vi "3.Dashboard.vi"() -> ()   [LabVIEW 2023]
uses:
  UnderAutomation.UniversalRobots/UnderAutomation.UniversalRobots.lvlib
  C:/Users/fg/Documents/UniversalRobots.vi/LabVIEW_2024/UnderAutomation.UniversalRobots/lib/UnderAutomation.UniversalRobots.dll
  LabVIEW_2024/UnderAutomation.UniversalRobots/lib/UnderAutomation.UniversalRobots.dll
panel:
  out "Dashboard":refnum<k24>
  out "UR Robot":refnum<k24>
  out "Connected":bool
  in  "Tab Control":enum32{"Connect to robot", "Commands", "State"}(tab)
  in  "Disconnect":bool
  in  "Test":bool
  in  "Key":string
  in  "Licensee":string
  in  "Connect":bool
  in  "IP":string caption="Robot IP Address"
  out "License state":string
  out "Connect error":string
  in  "Release brake":bool
  in  "Power Off":bool
  in  "Power On":bool
  out "Response":cluster{"Message":string, "Succeed":bool}
  in  "Program name":string
  in  "LoadProgram":bool
  in  "Get loaded program":bool
  out "Loaded program":string
  in  "Play":bool
  in  "Pause":bool
  in  "Stop":bool
  in  "Installation":string
  in  "Load installation":bool
  in  "Show popup":bool
  in  "message":string
  in  "Close popup":bool
  in  "Is program saved":bool
  out "IsSaved":bool
  in  "Get program state":bool
  out "Name":string
  out "State":i32(ring) items=["Stopped", "Playing", "Paused"]
  out "Value":T1
  in  "Get variable value":bool
  in  "name":string
  out "remote":bool
  in  "Is in remote control":bool
  in  "Get Serial number":bool
  in  "Get robot mode":bool
  out "Mode":i32(ring) items=["Disconnected"=0, "ConfirmSafety"=1, "Booting"=2, "PowerOff"=3, "PowerOn"=4, "Idle"=5, "BackDrive"=6, "Running"=7, "UpdatingFirmware"=8, "Other"=-1]
  in  "Get robot model":bool
  out "Model":i32(ring)=1 items=["UR5"=1, "UR10"=2, "UR3"=3, "UR16"=4]
  out "SN":string
  in  "stop":bool
  # "UnderAutomation"
  # "https://underautomation.com/universal-robots"
  # "+"
  # "LabVIEW demo app for remote control and monitoring of your Universal Robots cobot"
  # "Connect to robot"
  # "2. Ensure you have a trial or lifetime valid license"
  # "1. Set UR cobot address"
  # "This is a commercial library, you have a 30-day trial period. But you can use it forever if you buy a perpetual licence for your company (regardless of the number of robot, applications or developers)."
  # "If you have a license :"
  # "2. Connect to the robot"
  # "Power"
  # "Program"
  # "Installation"
  # "Popup"
  # "Remote control"
  # "Mode"
  # "Variable"
  # "S/N"
  # "Model"
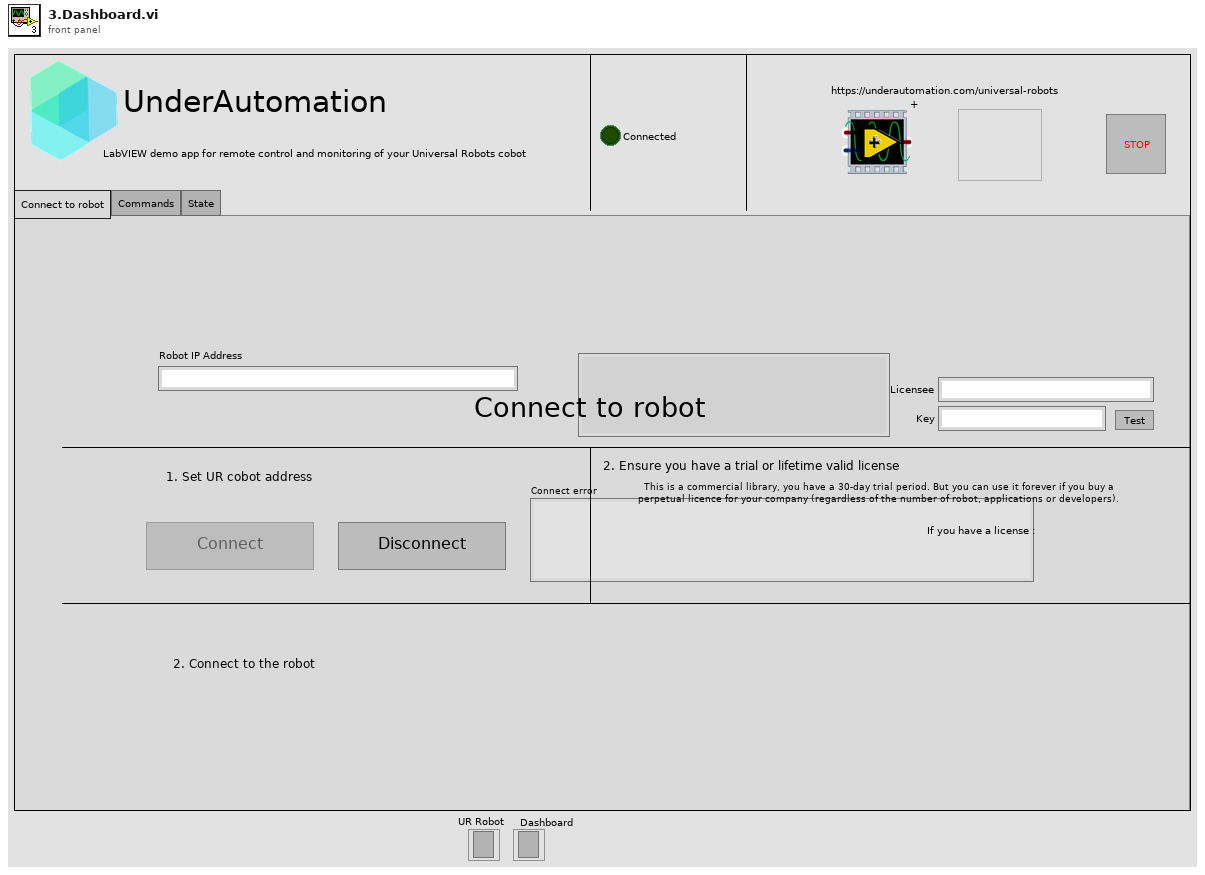
[diagram p1: front panel]
types:
  T1 = cluster{"Name":string, "Milliseconds":i32, "Type":i32, "BoolValue":bool, "FloatValue":sgl, "IntValue":i32, "StringValue":string, "PoseValue":cluster{"X":dbl, "Y":dbl, "Z":dbl, "Rx":dbl, "Ry":dbl, "Rz":dbl}}
  T2 = enum8{"Enabled", "Disabled", "Disabled and Grayed Out"}
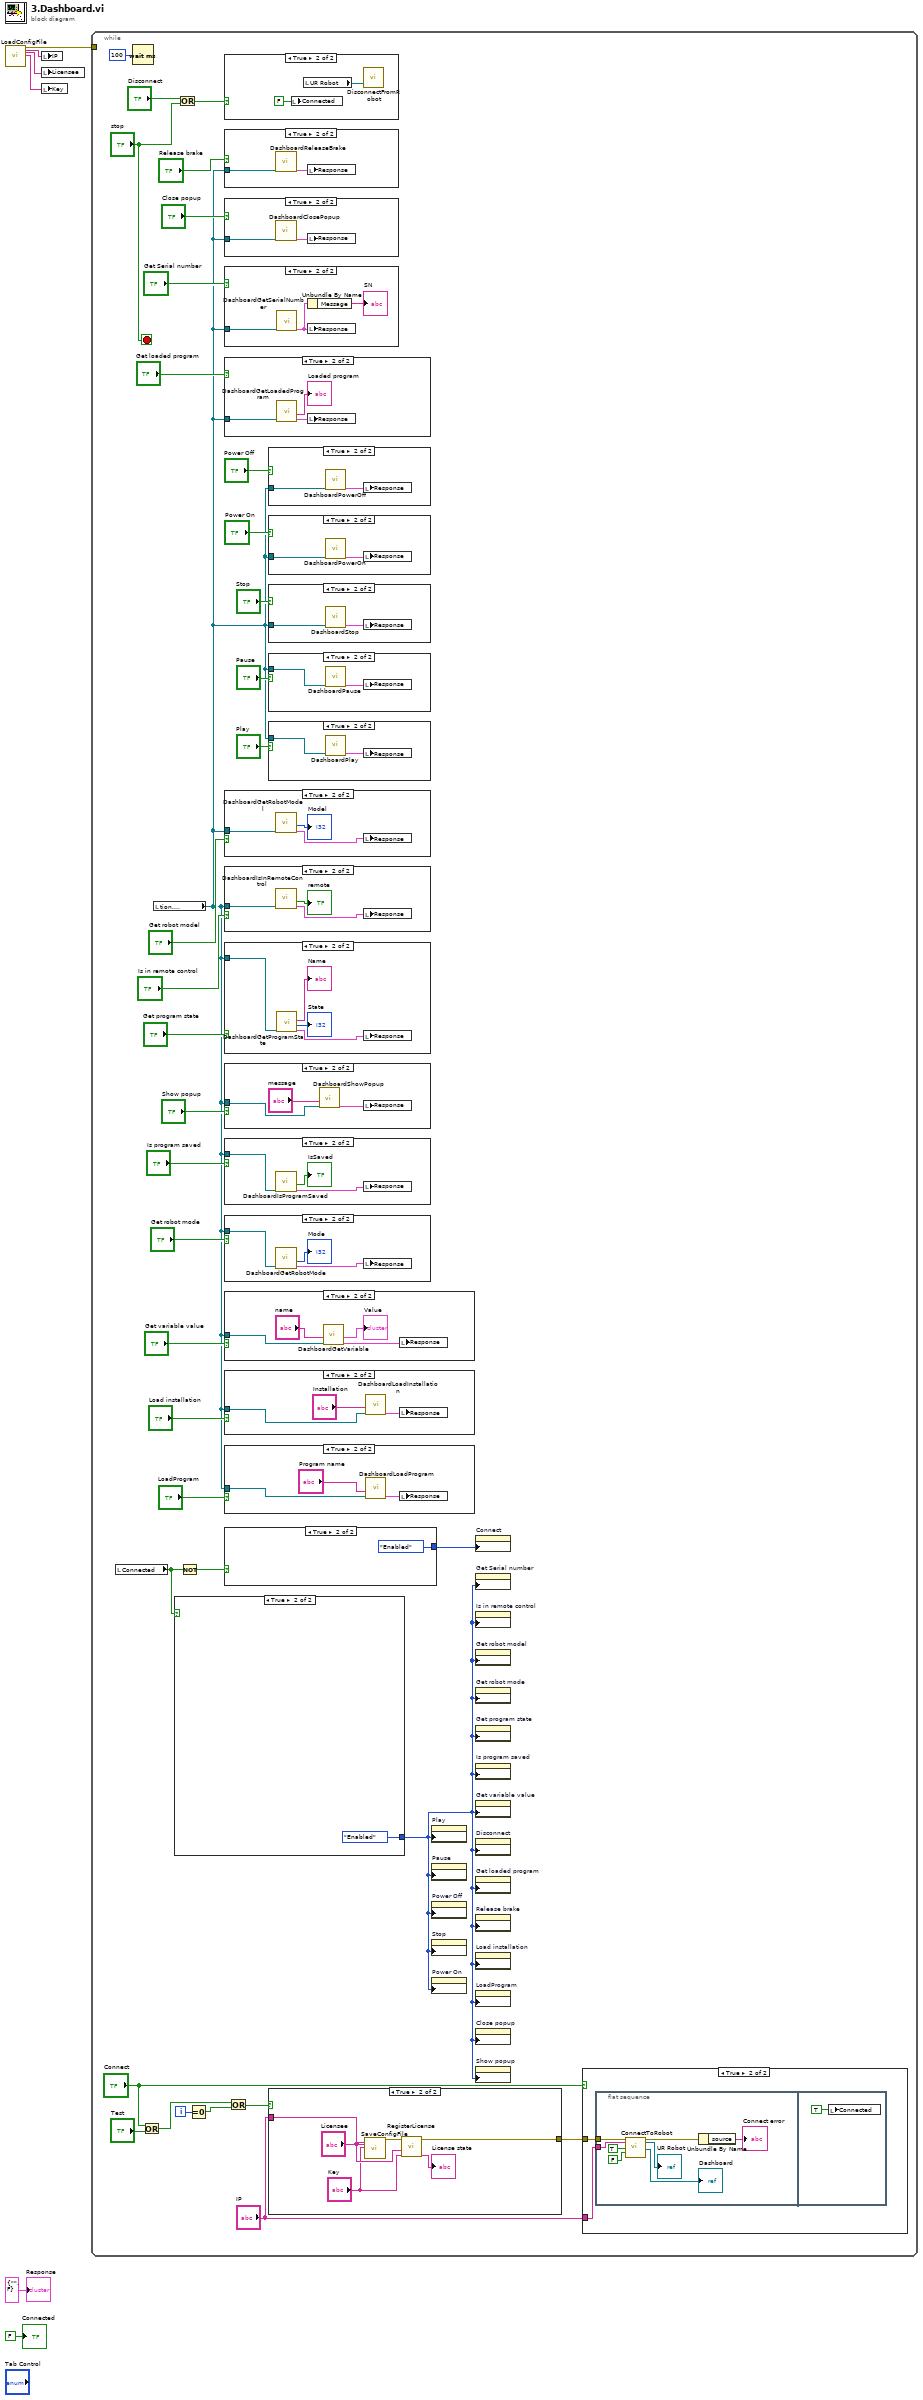
[diagram p0: block diagram]
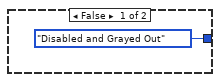
[diagram p20: hidden frame]
diagram:
  n1 = call "LoadConfigFile.vi"() -> ("error out"=w3:errorcluster, "IP"=w4:string, "Licensee"=w6:string, "Key"=w5:string)  [unwired: 22 in, 2 out]
  n2 = local write "IP"(w4) -> ()
  n3 = local write "Licensee"(w6) -> ()
  n4 = local write "Key"(w5) -> ()
  n5 = while {
    tunnel: w3 -> [_]
    i -> [w35]
    stop <- "stop" stop-if-true
    n6 = local read "Connected"() -> (w27:bool)
    n7 = Wait (ms)(milliseconds to wait=u32 100) -> ()  [unwired: 1 out]
    n8 = Or(x="Connect", y="Test") -> (x .or. y?=w33:bool)
    n9 = local read "Dashboard"() -> (w8:refnum<k24>)
    n10 = case shown="True" w27 {
      tunnel: [T2."Disabled and Grayed Out" ("Disabled") T2."Enabled" ("Disabled")] -> w7
      frame False {
      }
      frame True {
      }
    }
    n11 = Or(x="Disconnect", y="stop") -> (x .or. y?=w39:bool)
    n12 = Not(x=w27) -> (.not. x?=w29:bool)
    n13 = Equal To 0?(x=w35) -> (x = 0?=w34:bool)
    n14 = case shown="True" w39 {
      frame False {
      }
      frame True {
        n15 = local write "Connected"(FALSE ("Connected")) -> ()
        n16 = local read "UR Robot"() -> (w114:refnum<k24>)
        n17 = call "DisconnectFromRobot.vi"("UR Robot"=w114) -> ()  [unwired: 2 in, 1 out]
      }
    }
    n18 = case shown="True" "Release brake" {
      tunnel: w8 -> [_ w85]
      frame False {
      }
      frame True {
        n19 = call "DashboardReleaseBrake.vi"("Dashboard"=w85) -> ("Response"=w86:cluster{"Message":string, "Succeed":bool})  [unwired: 9 in, 1 out]
        n20 = local write "Response"(w86) -> ()
      }
    }
    n21 = case shown="True" "Close popup" {
      tunnel: w8 -> [_ w66]
      frame False {
      }
      frame True {
        n22 = call "DashboardClosePopup.vi"("Dashboard"=w66) -> ("Response"=w65:cluster{"Message":string, "Succeed":bool})  [unwired: 9 in, 1 out]
        n23 = local write "Response"(w65) -> ()
      }
    }
    n24 = case shown="True" "Get Serial number" {
      tunnel: w8 -> [_ w64]
      frame False {
      }
      frame True {
        n25 = call "DashboardGetSerialNumber.vi"("Dashboard"=w64) -> ("Response"=w63:cluster{"Message":string, "Succeed":bool})  [unwired: 9 in, 1 out]
        n26 = Unbundle By Name(w63) -> ("Message"=→"SN":string)
        n27 = local write "Response"(w63) -> ()
      }
    }
    n28 = case shown="True" "Get loaded program" {
      tunnel: w8 -> [_ w75]
      frame False {
      }
      frame True {
        n29 = call "DashboardGetLoadedProgram.vi"("Dashboard"=w75) -> ("Response"=w74:cluster{"Message":string, "Succeed":bool}, "loaded program"=→"Loaded program":string)  [unwired: 8 in, 1 out]
        n30 = local write "Response"(w74) -> ()
      }
    }
    n31 = case shown="True" "Get robot model" {
      tunnel: w8 -> [_ w56]
      frame False {
      }
      frame True {
        n32 = call "DashboardGetRobotModel.vi"("Dashboard"=w56) -> ("Response"=w58:cluster{"Message":string, "Succeed":bool}, "Model"=→"Model":i32)  [unwired: 8 in, 1 out]
        n33 = local write "Response"(w58) -> ()
      }
    }
    n34 = case shown="True" "Is in remote control" {
      tunnel: w8 -> [_ w50]
      frame False {
      }
      frame True {
        n35 = call "DashboardIsInRemoteControl.vi"("Dashboard"=w50) -> ("Response"=w52:cluster{"Message":string, "Succeed":bool}, "remote"=→"remote":bool)  [unwired: 8 in, 1 out]
        n36 = local write "Response"(w52) -> ()
      }
    }
    n37 = case shown="True" "Get program state" {
      tunnel: w8 -> [_ w42]
      frame False {
      }
      frame True {
        n38 = call "DashboardGetProgramState.vi"("Dashboard"=w42) -> ("Response"=w45:cluster{"Message":string, "Succeed":bool}, "State"=→"State":i32, "Name"=→"Name":string)  [unwired: 7 in, 1 out]
        n39 = local write "Response"(w45) -> ()
      }
    }
    n40 = case shown="True" "Show popup" {
      tunnel: w8 -> [_ w69]
      frame False {
      }
      frame True {
        n41 = call "DashboardShowPopup.vi"("Dashboard"=w69, "message"="message") -> ("Response"=w68:cluster{"Message":string, "Succeed":bool})  [unwired: 8 in, 1 out]
        n42 = local write "Response"(w68) -> ()
      }
    }
    n43 = case shown="True" "Is program saved" {
      tunnel: w8 -> [_ w53]
      frame False {
      }
      frame True {
        n44 = call "DashboardIsProgramSaved.vi"("Dashboard"=w53) -> ("Response"=w55:cluster{"Message":string, "Succeed":bool}, "IsSaved"=→"IsSaved":bool)  [unwired: 7 in, 2 out]
        n45 = local write "Response"(w55) -> ()
      }
    }
    n46 = case shown="True" "Get robot mode" {
      tunnel: w8 -> [_ w59]
      frame False {
      }
      frame True {
        n47 = call "DashboardGetRobotMode.vi"("Dashboard"=w59) -> ("Response"=w61:cluster{"Message":string, "Succeed":bool}, "Mode"=→"Mode":i32)  [unwired: 8 in, 1 out]
        n48 = local write "Response"(w61) -> ()
      }
    }
    n49 = case shown="True" "Get variable value" {
      tunnel: w8 -> [_ w47]
      frame False {
      }
      frame True {
        n50 = call "DashboardGetVariable.vi"("Dashboard"=w47, "name"="name") -> ("Response"=w49:cluster{"Message":string, "Succeed":bool}, "Value"=→"Value":T1)  [unwired: 7 in, 1 out]
        n51 = local write "Response"(w49) -> ()
      }
    }
    n52 = case shown="True" "Load installation" {
      tunnel: w8 -> [_ w71]
      frame False {
      }
      frame True {
        n53 = call "DashboardLoadInstallation.vi"("Dashboard"=w71, "installation"="Installation") -> ("Response"=w72:cluster{"Message":string, "Succeed":bool})  [unwired: 8 in, 1 out]
        n54 = local write "Response"(w72) -> ()
      }
    }
    n55 = case shown="True" "LoadProgram" {
      tunnel: w8 -> [_ w84]
      frame False {
      }
      frame True {
        n56 = call "DashboardLoadProgram.vi"("Dashboard"=w84, "programName"="Program name") -> ("Response"=w83:cluster{"Message":string, "Succeed":bool})  [unwired: 8 in, 1 out]
        n57 = local write "Response"(w83) -> ()
      }
    }
    n58 = case shown="True" w29 {
      tunnel: [T2."Disabled and Grayed Out" ("Disabled") T2."Enabled" ("Disabled")] -> w28
      frame False {
      }
      frame True {
      }
    }
    n59 = Or(x=w33, y=w34) -> (x .or. y?=w32:bool)
    n60 = case shown="True" "Power Off" {
      tunnel: w8 -> [_ w87]
      frame False {
      }
      frame True {
        n61 = call "DashboardPowerOff.vi"("Dashboard"=w87) -> ("Response"=w88:cluster{"Message":string, "Succeed":bool})  [unwired: 9 in, 1 out]
        n62 = local write "Response"(w88) -> ()
      }
    }
    n63 = case shown="True" "Power On" {
      tunnel: w8 -> [_ w89]
      frame False {
      }
      frame True {
        n64 = call "DashboardPowerOn.vi"("Dashboard"=w89) -> ("Response"=w90:cluster{"Message":string, "Succeed":bool})  [unwired: 9 in, 1 out]
        n65 = local write "Response"(w90) -> ()
      }
    }
    n66 = case shown="True" "Stop" {
      tunnel: w8 -> [_ w77]
      frame False {
      }
      frame True {
        n67 = call "DashboardStop.vi"("Dashboard"=w77) -> ("Response"=w76:cluster{"Message":string, "Succeed":bool})  [unwired: 9 in, 1 out]
        n68 = local write "Response"(w76) -> ()
      }
    }
    n69 = case shown="True" "Pause" {
      tunnel: w8 -> [_ w79]
      frame False {
      }
      frame True {
        n70 = call "DashboardPause.vi"("Dashboard"=w79) -> ("Response"=w78:cluster{"Message":string, "Succeed":bool})  [unwired: 9 in, 1 out]
        n71 = local write "Response"(w78) -> ()
      }
    }
    n72 = case shown="True" "Play" {
      tunnel: w8 -> [_ w81]
      frame False {
      }
      frame True {
        n73 = call "DashboardPlay.vi"("Dashboard"=w81) -> ("Response"=w80:cluster{"Message":string, "Succeed":bool})  [unwired: 9 in, 1 out]
        n74 = local write "Response"(w80) -> ()
      }
    }
    n75 = case shown="True" w32 {
      tunnel: [errorcluster {"status"=FALSE, "code"=0, "source"=""} ("error out") w100] -> w31
      tunnel: "IP" -> [_ w97]
      frame False {
      }
      frame True {
        n76 = call "SaveConfigFile.vi"("IP"=w97, "Licensee"="Licensee", "Key"="Key") -> ("error out"=w96:errorcluster)  [unwired: 24 in]
        n77 = call "RegisterLicense.vi"("key"="Key", "licensee"="Licensee", "error in"=w96) -> ("State message"=→"License state":string, "error out"=w100:errorcluster)  [unwired: 5 in, 1 out]
      }
    }
    n78 = property on="Play" class="Bool"("DisabledEnum"=w7) -> ()  [unwired: 2 in, 2 out]
    n79 = property on="Pause" class="Bool"("DisabledEnum"=w7) -> ()  [unwired: 2 in, 2 out]
    n80 = property on="Power Off" class="Bool"("DisabledEnum"=w7) -> ()  [unwired: 2 in, 2 out]
    n81 = property on="Stop" class="Bool"("DisabledEnum"=w7) -> ()  [unwired: 2 in, 2 out]
    n82 = property on="Power On" class="Bool"("DisabledEnum"=w7) -> ()  [unwired: 2 in, 2 out]
    n83 = property on="Connect" class="Bool"("DisabledEnum"=w28) -> ()  [unwired: 2 in, 2 out]
    n84 = property on="Get Serial number" class="Bool"("DisabledEnum"=w7) -> ()  [unwired: 2 in, 2 out]
    n85 = property on="Is in remote control" class="Bool"("DisabledEnum"=w7) -> ()  [unwired: 2 in, 2 out]
    n86 = property on="Get robot model" class="Bool"("DisabledEnum"=w7) -> ()  [unwired: 2 in, 2 out]
    n87 = property on="Get robot mode" class="Bool"("DisabledEnum"=w7) -> ()  [unwired: 2 in, 2 out]
    n88 = property on="Get program state" class="Bool"("DisabledEnum"=w7) -> ()  [unwired: 2 in, 2 out]
    n89 = property on="Is program saved" class="Bool"("DisabledEnum"=w7) -> ()  [unwired: 2 in, 2 out]
    n90 = property on="Get variable value" class="Bool"("DisabledEnum"=w7) -> ()  [unwired: 2 in, 2 out]
    n91 = property on="Disconnect" class="Bool"("DisabledEnum"=w7) -> ()  [unwired: 2 in, 2 out]
    n92 = property on="Get loaded program" class="Bool"("DisabledEnum"=w7) -> ()  [unwired: 2 in, 2 out]
    n93 = property on="Release brake" class="Bool"("DisabledEnum"=w7) -> ()  [unwired: 2 in, 2 out]
    n94 = property on="Load installation" class="Bool"("DisabledEnum"=w7) -> ()  [unwired: 2 in, 2 out]
    n95 = property on="LoadProgram" class="Bool"("DisabledEnum"=w7) -> ()  [unwired: 2 in, 2 out]
    n96 = property on="Close popup" class="Bool"("DisabledEnum"=w7) -> ()  [unwired: 2 in, 2 out]
    n97 = property on="Show popup" class="Bool"("DisabledEnum"=w7) -> ()  [unwired: 2 in, 2 out]
    n98 = case shown="True" "Connect" {
      tunnel: w31 -> [_ w103]
      tunnel: "IP" -> [_ w102]
      frame False {
        (unwired) refnum<k24> refnum ("Dashboard")
      }
      frame True {
        n99 = flat-sequence {
          tunnel: w103 -> [w106]
          tunnel: w102 -> [w105]
          frame #0 {
            n100 = call "ConnectToRobot.vi"("error in"=w106, "ip"=w105, "Enable Dashboard"=TRUE ("Enable Primary Interface"), "Enable Primary Interface"=FALSE) -> ("error out"=w109:errorcluster, "UR Robot"=→"UR Robot":refnum<k24>, "Dashboard"=→"Dashboard":refnum<k24>)  [unwired: 10 in, 3 out]
            n101 = Unbundle By Name(w109) -> ("source"=→"Connect error":string)
          }
          frame #1 {
            n102 = local write "Connected"(TRUE ("Connected")) -> ()
          }
        }
      }
    }
  }
  "Connected" <- FALSE ("Connected")
  "Response" <- cluster{"Message":string, "Succeed":bool} {"Message"="", "Succeed"=FALSE} ("Response")
